vi "Update Info.vi"(8 "error in (no error)":errorcluster, 9 "Get All Info":bool, 11 "CIF_UI in":refnum<class "CIF_UI.lvclass">) -> (0 "error out":errorcluster, 1 "Info":string)   [LabVIEW 2021, in "CIF_UI.lvclass"]
uses:
  CIF_UI.lvclass
  CIF_UI.lvclass/CIF_UI.ctl
  CIFPluginManager/CIFPluginManager/gRPC/CIF_Manager_Client_Wrapper/CIFManagerClientWrapper.lvlib
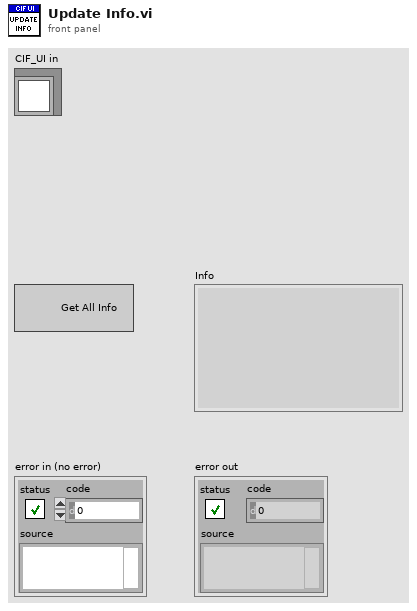
[diagram p1: front panel]
types:
  T1 = typedef "grpc-lvsupport-release.lvlib/grpcId.ctl" = u64
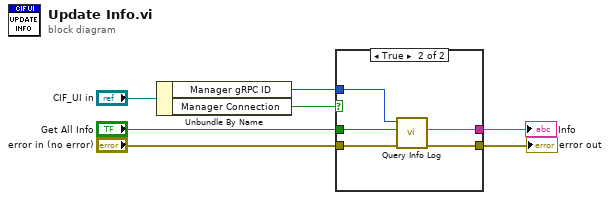
[diagram p0: block diagram]
diagram:
  n1 = Unbundle By Name("CIF_UI in") -> ("Manager gRPC ID"=w3:T1, "Manager Connection"=w1:bool)
  n2 = case shown="True" w1 {
    tunnel: "Get All Info" -> [_ w13]
    tunnel: [w8 w9] -> w5
    tunnel: [_ w12] -> w4
    tunnel: w3 -> [_ w11]
    tunnel: "error in (no error)" -> [w8 w10]
    frame False {
    }
    frame True {
      n3 = call "Query Info Log.vi"("error in"=w10, "query_all"=w13, "gRPC ID in"=w11) -> ("error out"=w9:errorcluster, "Info"=w12:string)  [unwired: 6 in, 1 out]
    }
  }
  "error out" <- w5
  "Info" <- w4
